vi "Write Samples per Fetch.vi"(8 "error in (no error)":errorcluster, 10 "Samples per Loop":i32=100, 11 "Fetch Waveforms CFG in":refnum<class "Fetch Waveforms CFG.lvclass">) -> (0 "error out":errorcluster, 3 "Fetch Waveforms CFG out":refnum<class "Fetch Waveforms CFG.lvclass">)   [LabVIEW 2023, in "PXIe-4353.lvlib" / "Fetch Waveforms CFG.lvclass"]
uses:
  Fetch Waveforms CFG.lvclass
  Fetch Waveforms CFG.lvclass/Fetch Waveforms CFG.ctl
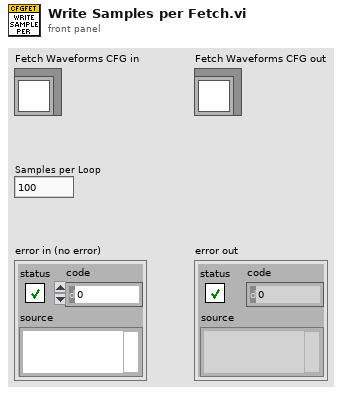
[diagram p1: front panel]
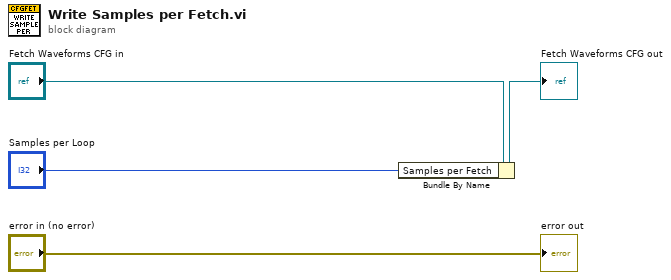
[diagram p0: block diagram]
diagram:
  n1 = Bundle By Name(cluster="Fetch Waveforms CFG in", "Samples per Fetch"="Samples per Loop") -> (→"Fetch Waveforms CFG out":refnum<class "Fetch Waveforms CFG.lvclass">)
  "error out" <- "error in (no error)"
